vi "SRLatch.vi"(1 "On":bool, 2 "Off":bool, 3 "Initial":bool) -> (0 "Output":bool)   [LabVIEW 2018]
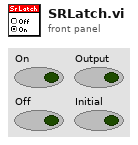
[diagram p1: front panel]
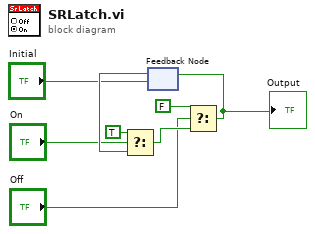
[diagram p0: block diagram]
diagram:
  n1 = feedback #1("Initial") -> (w7:bool)
  n2 = Select(t=TRUE, s="On", f=w7) -> (s? t:f=w8:bool)
  n3 = Select(t=FALSE, s="Off", f=w8) -> (s? t:f=w2:bool)
  "Output" <- w2
  n4 = feedback-in #1(w2) -> ()
